vi "Attach Observer.vi"(8 "error in":errorcluster, 10 "Observer":refnum<queue>, 11 "Data Subject in":refnum<class "Publisher.lvclass">) -> (0 "error out":errorcluster, 3 "Data Subject out":refnum<class "Publisher.lvclass">)   [LabVIEW 2014, in "Publisher.lvclass"]
uses:
  Publisher.lvclass
  Data/Data.lvclass
  Publisher.lvclass/Publisher.ctl
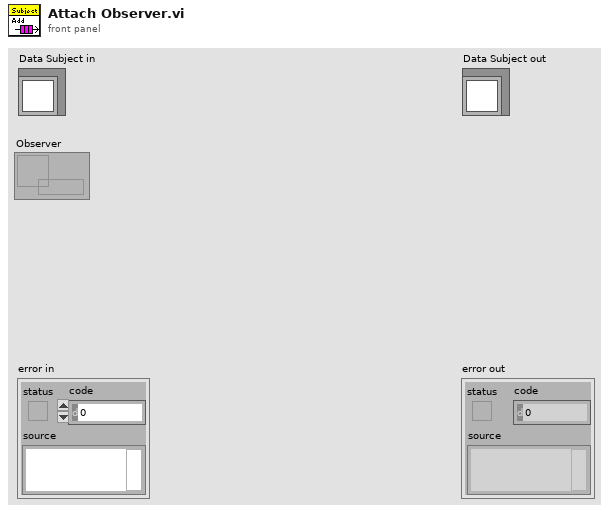
[diagram p1: front panel]
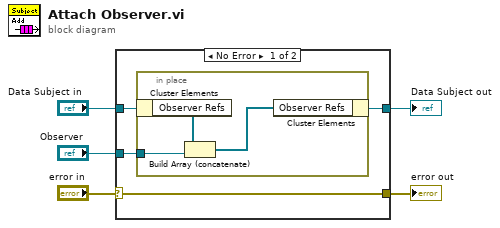
[diagram p0: block diagram]
diagram:
  n1 = case shown="No Error" "error in" {
    selector: "error in" -> [w6 w14]
    tunnel: [w6 w14] -> w4
    tunnel: [w7 w13] -> w2
    tunnel: "Data Subject in" -> [w9 w13]
    tunnel: "Observer" -> [w8 _]
    frame No Error {
      n2 = in-place {
        in-place-border: w8 -> [w11]
        n3 = in-place-cluster #1(w9) -> ("Observer Refs"=w12:refnum<queue>[])
        n4 = Build Array (concatenate)(w12, w11) -> (w10:refnum<queue>[])
        n5 = in-place-cluster #1("Observer Refs"=w10) -> (w7:refnum<class "Publisher.lvclass">)
      }
    }
    frame Error {
    }
  }
  "error out" <- w4
  "Data Subject out" <- w2
